vi "generate file data.vi"(8 "error in":errorcluster, 11 "file information":T1) -> (0 "error out":errorcluster, 3 "file format":T6)   [LabVIEW 2013, in "PLConfigurationSerializer.lvlib"]
uses:
  PLConfigurationSerializer.lvlib
  file format.ctl
  1_0_0_0 format.ctl
  system hierarchy.ctl
  target hierarchy.ctl
  engine hierarchy.ctl
  configuration database.ctl
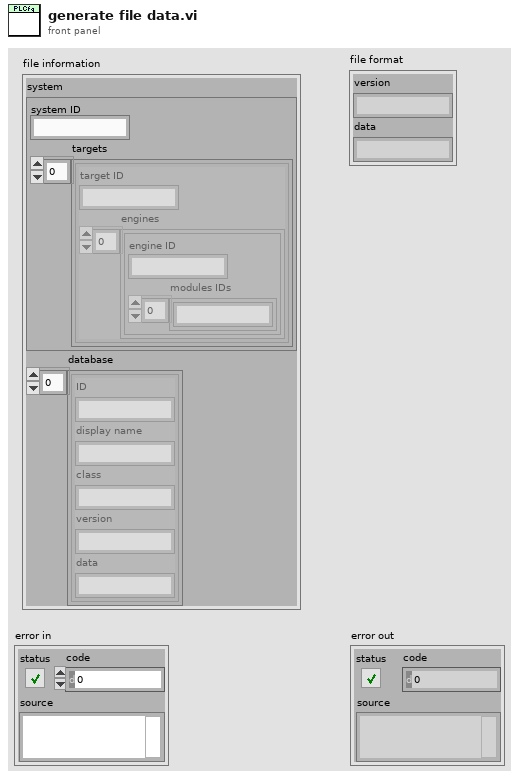
[diagram p1: front panel]
types:
  T1 = typedef "PLConfigurationSerializer.lvlib/1_0_0_0 format.ctl" = cluster{"system":T2, "database":T5[]}
  T2 = typedef "PLConfigurationSerializer.lvlib/system hierarchy.ctl" = cluster{"system ID":string, "targets":T3[]}
  T3 = typedef "PLConfigurationSerializer.lvlib/target hierarchy.ctl" = cluster{"target ID":string, "engines":T4[]}
  T4 = typedef "PLConfigurationSerializer.lvlib/engine hierarchy.ctl" = cluster{"engine ID":string, "modules IDs":string[]}
  T5 = typedef "PLConfigurationSerializer.lvlib/configuration database.ctl" = cluster{"ID":string, "display name":string, "class":string, "version":string, "data":string}
  T6 = typedef "PLConfigurationSerializer.lvlib/file format.ctl" = cluster{"version":string, "data":string}
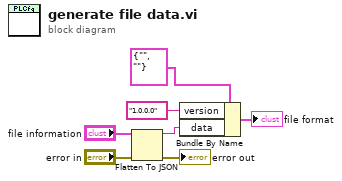
[diagram p0: block diagram]
diagram:
  n1 = Flatten To JSON(anything="file information", error in (no error)="error in") -> (JSON string=w1:string, 11:→"error out":errorcluster)  [unwired: 1 in]
  n2 = Bundle By Name(cluster=T6 {"version"="", "data"=""} ("file format"), "version"="1.0.0.0", "data"=w1) -> (→"file format":T6)
